vi "day 3 task 2.vi"() -> ()   [LabVIEW 2019]
uses:
  672666e8-34fd-4b20-9318-adf5440ec777.vi
  8b16236f-c8de-4b08-a6c4-6a4b4e7bf06e.vi
  b6a642f0-c0f9-4ebb-a633-59b7cc25d075.vi
panel:
  out "sum(answer)":u64
  out "Priorities of badge item":u8[][](array[numeric])
  out "error log":string[](array[string])
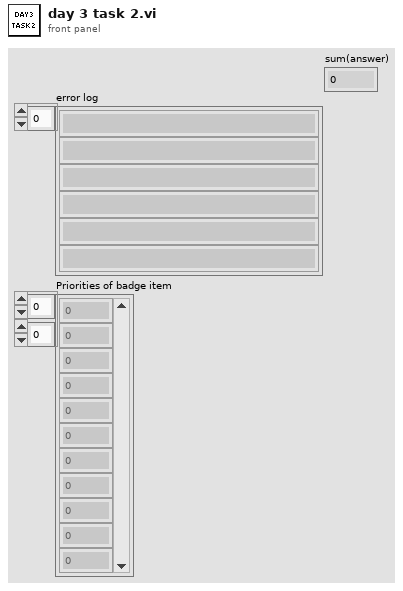
[diagram p1: front panel]
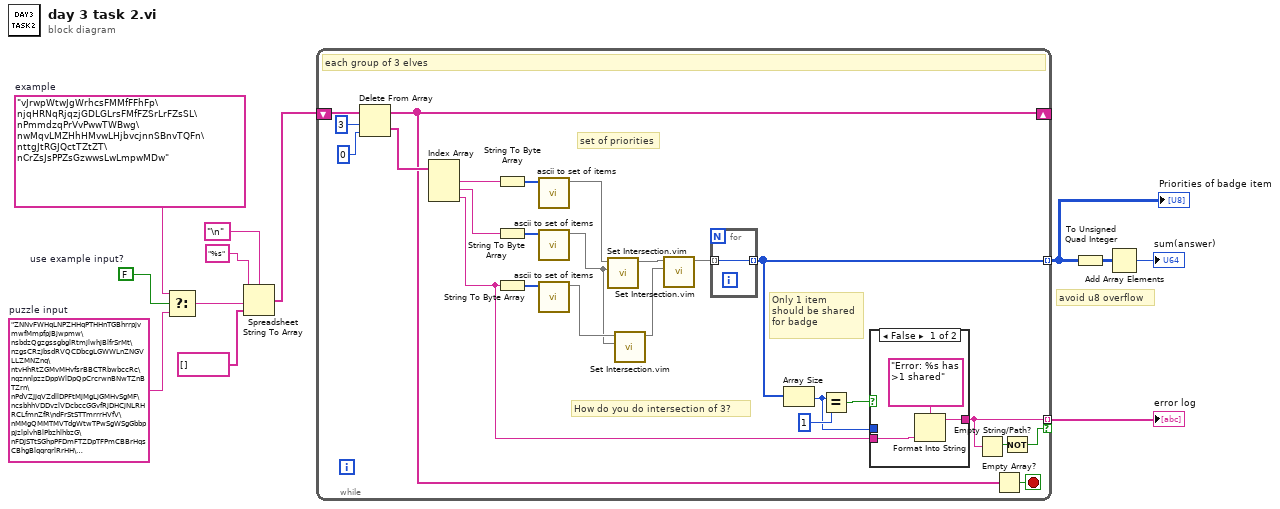
[diagram p0: block diagram]
diagram:
  w7 = FALSE  # use example input?
  w8 = "ZNNvFWHqLNPZHHqPTHHnTGBhrrpjvmwfMmpfpjBjwpmw\nsbdzQgzgssgbglRtmjlwhjBlfrSrMt\nzgsCRzJbsdRVQCDbcgLGWWLnZNGVLLZMNZnq\ntvHhRtZGMvMHvfsrBBCTRbwbccRc\nqznnlpzzDppWlDpQpCrcrwnBNwTZnBTZrn\nPdVZJJqVZdllDPFtMjMgLjGMHvSgMF\ncsbhhVDDvzlVDcbccGGvfRjDHCjNLRHRCLfmnZfR\ndFrStSTTmrrrHVfV\nMMgQMMTMVTdgWtwTPwSgWSgGbbppJzlplvhBlPbzhlhbzG\nFDJSTtSGhpPFDmFTZDpTFPmCBBrHqsCBhgBlqqrqrlRrHH\ndQwMtfdzVwWfwctwnfnQCHllzRrsNzrrgNlCgqsr\nfLfQnVjfwQfMdfvfnVvWDvtJPFGDpvZGbZpmbSPP\nTzzCrJcDrTDdLDCJDvGNPCFqlZWlvNvWpq\nRRHfjsQBFsjgjBQsWqGpNvZQqQlPPQPN\nVnHBnRVssnnjsSfBwbMSrrbTwJTcwSDF\nHJCgHCCFFFVGJWTlbqDdlqTDDpgl\ncZccSmLrfZcrmmzSQftdpDtTHdbQ..."  # puzzle input
  w9 = "vJrwpWtwJgWrhcsFMMfFFhFp\njqHRNqRjqzjGDLGLrsFMfFZSrLrFZsSL\nPmmdzqPrVvPwwTWBwg\nwMqvLMZHhHMvwLHjbvcjnnSBnvTQFn\nttgJtRGJQctTZtZT\nCrZsJsPPZsGzwwsLwLmpwMDw"  # example
  # "avoid u8 overflow"
  n1 = Select(t=w9, s=w7, f=w8) -> (s? t:f=w6:string)
  n2 = Spreadsheet String To Array(delimiter (Tab)="\n", format string="%s", spreadsheet string=w6, array type (2D Dbl)=string[] []) -> (array=w1:string[])
  n3 = while {
    tunnel: [w30] -> w3 mode=indexing
    tunnel: [w34] -> w5 mode=indexing if=w33
    shift-right: [w13] -> _
    shift-left: w1 -> [w25]
    stop <- w14 stop-if-true
    # "How do you do intersection of 3?"
    # "Only 1 item\nshould be shared\nfor badge"
    # "set of priorities"
    # "each group of 3 elves"
    n4 = Delete From Array(array=w25, length=3, index=0) -> (deleted portion=w24:string[], array with subset deleted=w13:string[])
    n5 = Index Array(array=w24) -> (element #1=w23:string, element #2=w22:string, element #3=w15:string)  [unwired: 3 in]
    n6 = String To Byte Array(string=w23) -> (unsigned byte array=w28:u8[])
    n7 = String To Byte Array(string=w22) -> (unsigned byte array=w29:u8[])
    n8 = String To Byte Array(string=w15) -> (unsigned byte array=w21:u8[])
    n9 = call "ascii to set of items.vi"("ascii bytes"=w28) -> ("set out"=w37:set{u8})  [unwired: 10 in]
    n10 = call "ascii to set of items.vi"("ascii bytes"=w29) -> ("set out"=w19:set{u8})  [unwired: 10 in]
    n11 = call "ascii to set of items.vi"("ascii bytes"=w21) -> ("set out"=w20:set{u8})  [unwired: 10 in]
    n12 = call "Set Intersection.vim"("set 2"=w19, "set 1"=w37) -> ("intersection"=w17:set{u8})  [unwired: 9 in]
    n13 = call "Set Intersection.vim"("set 2"=w19, "set 1"=w20) -> ("intersection"=w18:set{u8})  [unwired: 9 in]
    n14 = call "Set Intersection.vim"("set 2"=w18, "set 1"=w17) -> ("intersection"=w16:set{u8})  [unwired: 9 in]
    n15 = for {
      tunnel: [w41] -> w30 mode=indexing
      tunnel: w16 -> [w41] mode=indexing
    }
    n16 = Array Size(array=w30) -> (size(s)=w31:i32)
    n17 = Equal?(x=w31, y=1) -> (x = y?=w35:bool)
    n18 = case shown="False" w35 {
      tunnel: [w39 _] -> w34
      tunnel: w31 -> [_ _]
      tunnel: w15 -> [w38 _]
      frame False {
        n19 = Format Into String(format string="Error: %s has >1 shared", w38) -> (resulting string=w39:string)  [unwired: 2 in, 1 out]
      }
      frame True {
      }
    }
    n20 = Empty String/Path?(string/path=w34) -> (empty?=w32:bool)
    n21 = Empty Array?(array=w13) -> (empty?=w14:bool)
    n22 = Not(x=w32) -> (.not. x?=w33:bool)
  }
  "error log" <- w5
  "Priorities of badge item" <- w3
  n23 = To Unsigned Quad Integer(1:w3) -> (0:w4:u64[][])
  n24 = Add Array Elements(numeric array=w4) -> (sum=→"sum(answer)":u64)
